vi "Field_C action on update.vi"(4 "Overall status in":T4) -> (0 "Overall status Out":T4, 1 "Command out":T3=enum."Set field")   [LabVIEW 2024, in "Magnet module.lvlib"]
doc: "Evaluates next state machine action at the end of regular check.\nIf field is not at desired value, but reached the closest target it sets new target with new ramp."
uses:
  Magnet module.lvlib
  ctl/RampingOutput.ctl
  ctl/Magnet Orders.ctl
  ctl/Magnet mode.ctl
  ctl/Magnet mode public.ctl
  ctl/SetField data.ctl
  ctl/Overall status.ctl
  ctl/Actual magnet state.ctl
  ctl/Magnet config constants.ctl
  <instrlib>/SMS drivers/Public/PSU Status.ctl
  <instrlib>/SMS drivers/Cryogenic Ltd SMSXXX.lvlib
panel:
  out "error out":errorcluster
  in  "Error In":errorcluster
  in  "PSU Status In":T1 {"Trip Current" format="%.3f"; "Trip Field" format="%.4f"; "Voltage" format="%.2f"; "Field Constant" format="%.6f"; "MID Setpoint (T)" format="%.4f"; "MID Setpoint (A)" format="%.3f"; "MAX Setpoint (T)" format="%.4f"; "MAX Setpoint (A)" format="%.3f"; "Heater Voltage" format="%.2f"; "V Limit (V)" format="%.2f"; "Ramp Rate (A/s)" format="%.3f"; "Output (A)" format="%.3f"; "Output (T)" format="%.4f"; "Persistent Current" format="%.3f"; "Persistent Field" format="%.4f"}
  in  "Magnet Config Constants":T2={"Switch resistant [K]"=5.0, "Switch superconducting [K]"=4.0, "First stage critical temperature [K]"=50.0, "Second stage critical temperature [K]"=5.0, "Inner magnet critical temperature [K]"=6.0, "Outer magnet critical temperature [K]"=5.0, "Field Constant [T/A]"=0.14911, "Maximum Current [A]"=107.3, "Maximum field [T]"=16.0, "Maximum source ramp [A/s]"=0.5, "Source precision [T]"=2e-05, "Ramp limits [A/s]"=[0.0506, 0.038, 0.0285, 0.0213, 0.0104], "Field limits [T]"=[3.0, 9.6, 13.3, 15.5, 16.0], "SMS"="", "LSC218"=""}
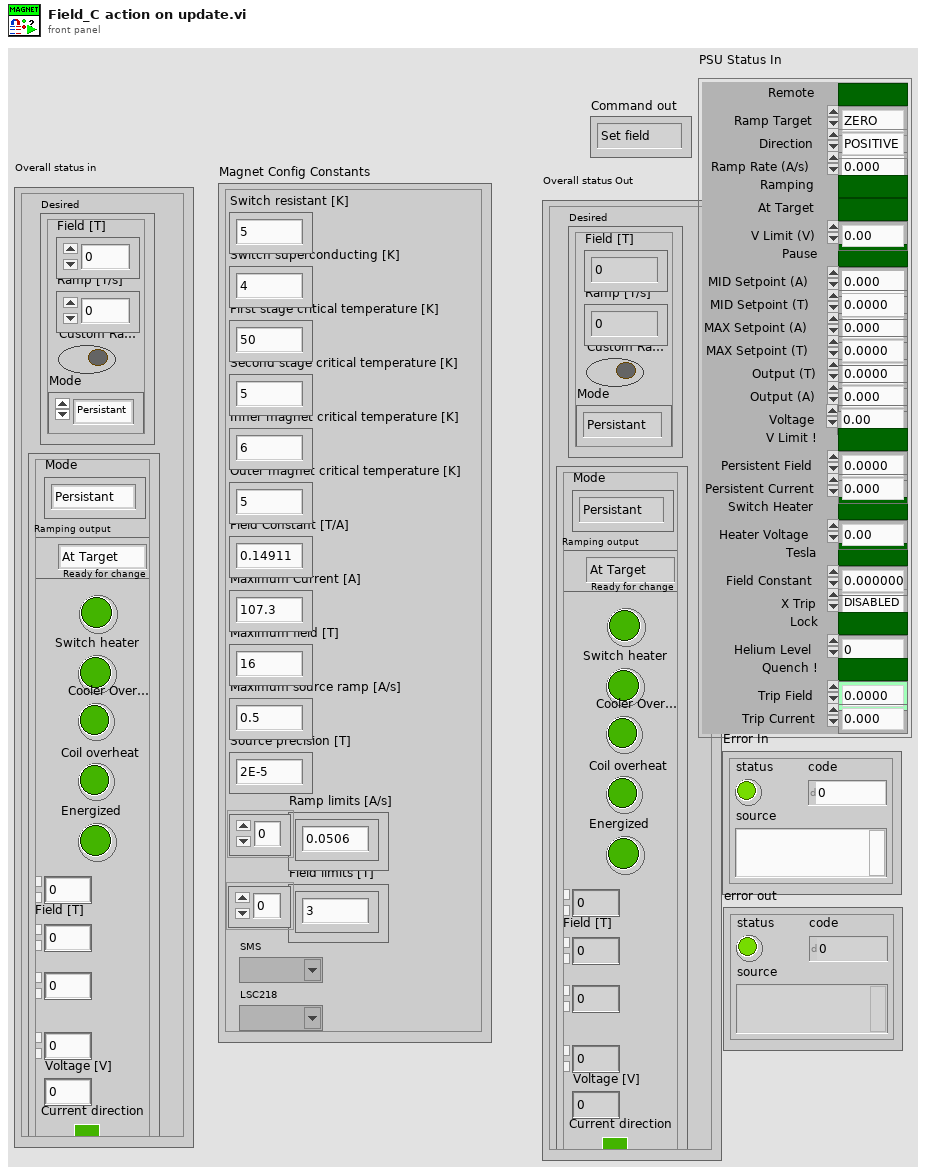
[diagram p1: front panel]
types:
  T1 = typedef "Cryogenic Ltd SMSXXX.lvlib/PSU Status.ctl" = cluster{"Ramp Target":enum16{"ZERO", "MID", "MAX"}, "Pause":bool, "Switch Heater":bool, "Persistent Field":dbl, "Persistent Current":dbl, "Tesla":bool, "Output (T)":dbl, "Output (A)":dbl, "X Trip":enum16{"DISABLED", "ENABLED", "ACTIVE"}, "Ramp Rate (A/s)":dbl, "V Limit (V)":dbl, "Heater Voltage":dbl, "MAX Setpoint (A)":dbl, "MAX Setpoint (T)":dbl, "MID Setpoint (A)":dbl, "MID Setpoint (T)":dbl, "Lock":bool, "Field Constant":dbl, "Remote":bool, "Direction":enum16{"POSITIVE", "NEGATIVE", "OPEN", "UNIPOLAR"}, "Helium Level":u16, "Quench !":bool, "Voltage":dbl, "V Limit !":bool, "Ramping":bool, "At Target":bool, "Trip Field":dbl, "Trip Current":dbl}
  T2 = typedef "Magnet module.lvlib/Magnet config constants.ctl" = cluster{"Switch resistant [K]":dbl, "Switch superconducting [K]":dbl, "First stage critical temperature [K]":dbl, "Second stage critical temperature [K]":dbl, "Inner magnet critical temperature [K]":dbl, "Outer magnet critical temperature [K]":dbl, "Field Constant [T/A]":dbl, "Maximum Current [A]":dbl, "Maximum field [T]":dbl, "Maximum source ramp [A/s]":dbl, "Source precision [T]":dbl, "Ramp limits [A/s]":dbl[], "Field limits [T]":dbl[], "SMS":refnum<visa-resource-name>, "LSC218":refnum<visa-resource-name>}
  T3 = typedef "Magnet module.lvlib/Magnet Orders.ctl" = enum16{"Ignore", "Connect", "Update", "Switch mode", "Set field", "Stop ramping", "Equalize output", "Zero output", "Flip polarity", "Blackout", "Set timer", "Eval temperatures", "Disconnect"}
  T4 = typedef "Magnet module.lvlib/Overall status.ctl" = cluster{"Desired":T5, "Actual":T7}
  T5 = typedef "Magnet module.lvlib/SetField data.ctl" = cluster{"Field [T]":dbl, "Ramp [T/s]":dbl, "Custom Ramp?":bool, "Mode":T6}
  T6 = typedef "Magnet module.lvlib/Magnet mode public.ctl" = enum16{"Persistant", "Ramping"}
  T7 = typedef "Magnet module.lvlib/Actual magnet state.ctl" = cluster{"Mode":T8, "Ramping output":T9, "Ready for change":bool, "Switch heater":bool, "Cooler Overheat":bool, "Coil overheat":bool, "Energized":bool, "Output [T]":dbl, "Field [T]":dbl, "Ramp[T/s]":dbl, "Switch\ntemperature [K]":dbl, "Voltage [V]":dbl, "Current direction":bool}
  T8 = typedef "Magnet module.lvlib/Magnet mode.ctl" = enum16{"Persistant", "Switching", "Ramping", "Quenched"}
  T9 = typedef "Magnet module.lvlib/RampingOutput.ctl" = enum16{"At Target", "Go up", "Go down"}
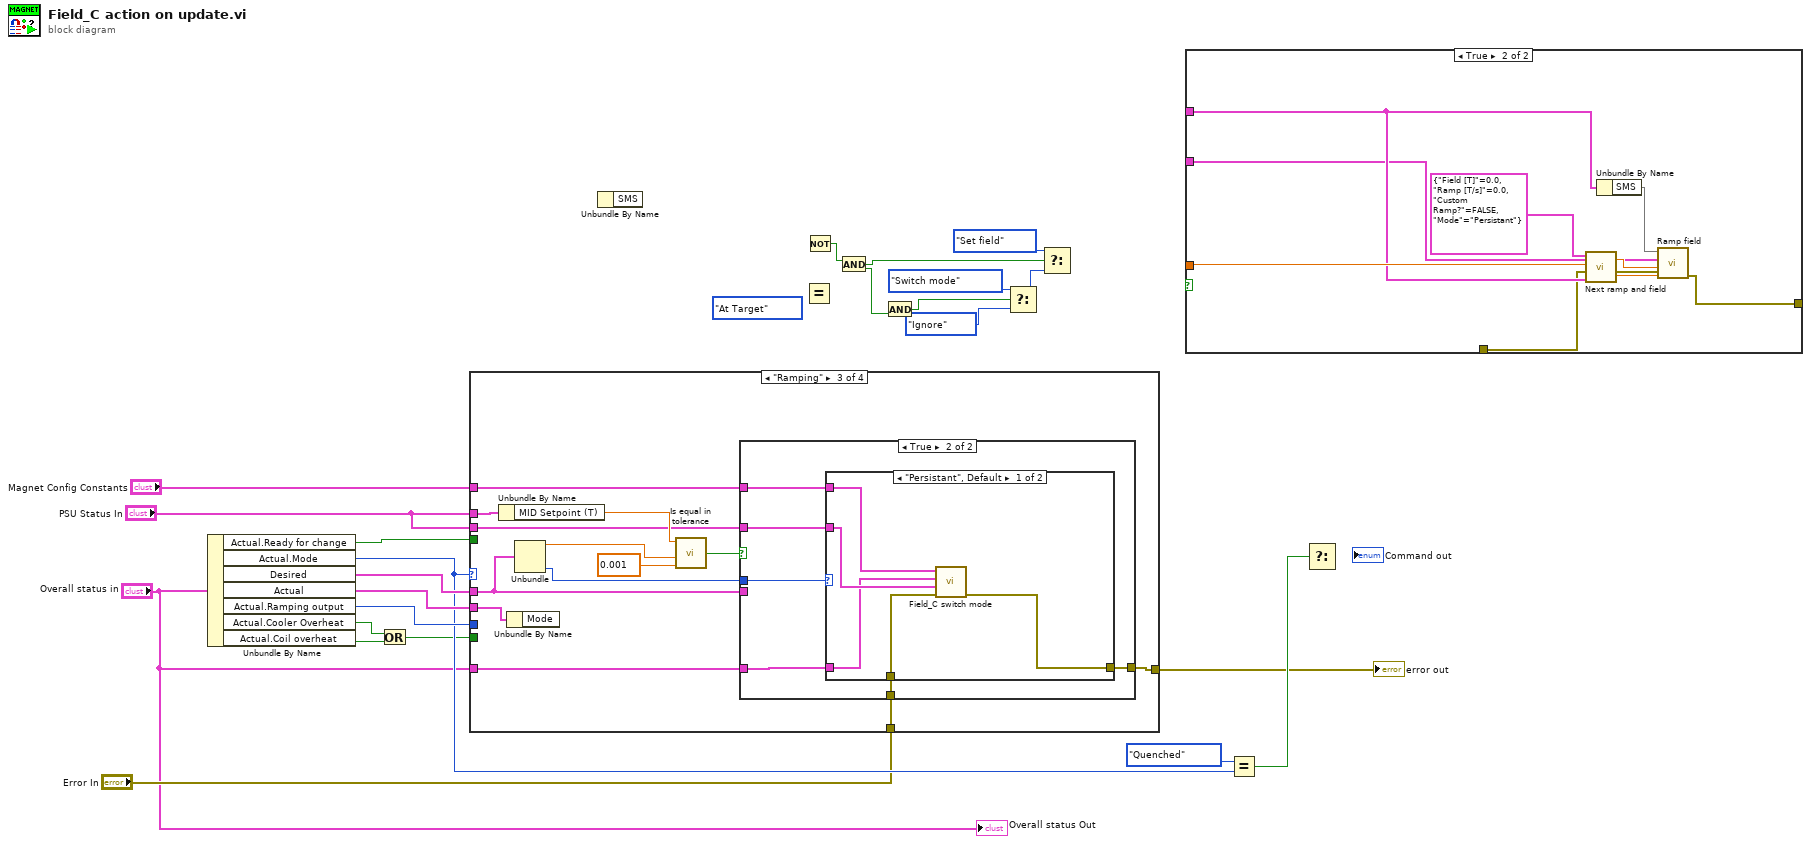
[diagram p0: block diagram]
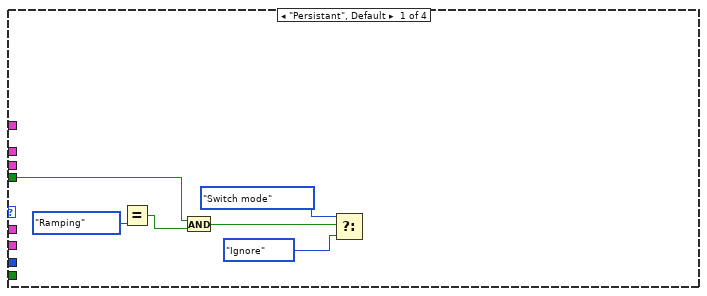
[diagram p3: hidden frame]
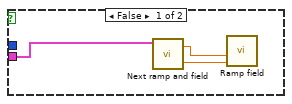
[diagram p5: hidden frame]
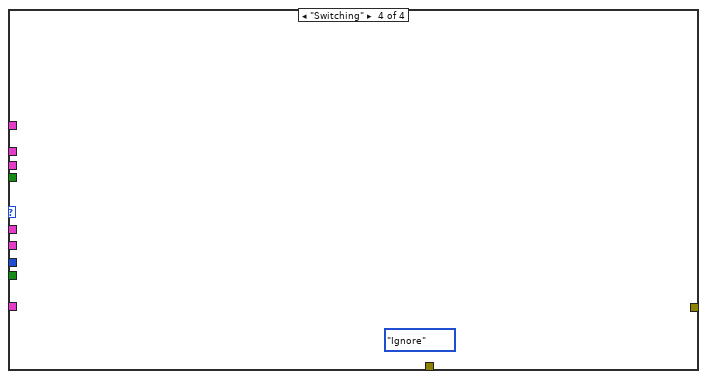
[diagram p7: hidden frame]
diagram:
  (unwired) RampingOutput."At Target" ("x")
  n1 = Unbundle By Name("Overall status in") -> ("Actual.Ready for change"=w15:bool, "Actual.Mode"=w20:T8, "Desired"=w22:T5, "Actual"=w23:T7, "Actual.Ramping output"=w21:T9, "Actual.Cooler Overheat"=w17:bool, "Actual.Coil overheat"=w16:bool)
  n2 = Or(x=w17, y=w16) -> (x .or. y?=w14:bool)
  n3 = case shown="\"Ramping\"" w20 {
    tunnel: w23 -> [_ _ w40 _]
    tunnel: w22 -> [_ _ w41 _]
    tunnel: w21 -> [_ _ _ _]
    tunnel: w15 -> [w24 _ _ _]
    tunnel: w14 -> [_ _ _ _]
    tunnel: "Magnet Config Constants" -> [_ _ w37 _]
    tunnel: "PSU Status In" -> [_ _ w36 _]
    tunnel: [_ _ w33 _] -> w4
    tunnel: "Error In" -> [_ _ w34 _]
    tunnel: "PSU Status In" -> [_ _ w35 _]
    tunnel: "Overall status in" -> [_ _ w32 _]
    frame "Persistant", Default {
      n4 = Equal?(y=Magnet_mode_public."Ramping" ("Mode")) -> (x=w27:T6, x = y?=w25:bool)
      n5 = And(x=w24, y=w25) -> (x .and. y?=w28:bool)
      n6 = Select(t=Magnet_Orders."Switch mode" ("Command out"), s=w28, f=Magnet_Orders."Ignore" ("Command out")) -> (s? t:f=w29:T3)
    }
    frame "Quenched" {
      # "If quenched, do nothing or just set current to zero"
    }
    frame "Ramping" {
      n7 = Unbundle By Name(w36) -> ("MID Setpoint (T)"=w43:dbl)
      n8 = Unbundle By Name(w40) -> ()  [unwired: 1 out]
      n9 = Unbundle(w41) -> ("Field [T]"=w42:dbl, "Mode"=w38:T6)  [unwired: 2 out]
      n10 = call "Is equal in tolerance.vi"("Absolut tolerance"=0.001, "Reference value"=w42, "Input value"=w43) -> ("Is in range"=w39:bool)  [unwired: 1 in]
      n11 = case shown="True" w39 {
        tunnel: w41 -> [w45 _]
        tunnel: w38 -> [_ w53]
        tunnel: w37 -> [_ w52]
        tunnel: w35 -> [_ w51]
        tunnel: w34 -> [_ w50]
        tunnel: [_ w49] -> w33
        tunnel: w32 -> [_ w48]
        frame False {
          n12 = call "Next ramp and field.vi"("Desired"=w45) -> ("Ramp to set [A/s]"=w47:dbl, "Field to set [T]"=w46:dbl)  [unwired: 3 in]
          n13 = call "Ramp field.vi"("Ramp to set [A/s]"=w47, "Field to set [T]"=w46) -> ()  [unwired: 6 in, 4 out]
        }
        frame True {
          n14 = case shown="\"Persistant\", Default" w53 {
            tunnel: w52 -> [w54 _]
            tunnel: w51 -> [w58 _]
            tunnel: w50 -> [w57 _]
            tunnel: [w56 _] -> w49
            tunnel: w48 -> [w55 _]
            frame "Persistant", Default {
              n15 = call "Field_C switch mode.vi"("error in (no error)"=w57, "PSU Status"=w58, "Overall status in"=w55, "Magnet Constants"=w54) -> ("error out"=w56:errorcluster)  [unwired: 5 in, 2 out]
            }
            frame "Ramping" {
            }
          }
        }
      }
    }
    frame "Switching" {
      (unwired) Magnet_Orders."Ignore" ("Command out")
    }
  }
  "error out" <- w4
  n16 = Unbundle By Name() -> ()  [unwired: 1 in, 1 out]
  n17 = Equal?() -> ()  [unwired: 2 in, 1 out]
  n18 = Not() -> (.not. x?=w9:bool)  [unwired: 1 in]
  n19 = And(x=w9) -> (y=w13:bool, x .and. y?=w10:bool)
  n20 = And(y=w13) -> (x .and. y?=w12:bool)  [unwired: 1 in]
  n21 = Select(t=Magnet_Orders."Switch mode", s=w12, f=Magnet_Orders."Ignore" ("Command out")) -> (s? t:f=w11:T3)
  n22 = Select(t=Magnet_Orders."Set field" ("Command out"), s=w10, f=w11) -> ()  [unwired: 1 out]
  n23 = case shown="True" {
    selector: _ -> [_ _]
    tunnel: _ -> [_ w66]
    tunnel: _ -> [_ w64]
    tunnel: _ -> [_ w62]
    tunnel: [w59 w60] -> _
    tunnel: [w59 w61] -> _
    frame False {
    }
    frame True {
      n24 = call "Next ramp and field.vi"("Magnet Constants in"=w64, "Actual field [T]"=w66, "Desired"=T5 {"Field [T]"=0.0, "Ramp [T/s]"=0.0, "Custom Ramp?"=FALSE, "Mode"=enum."Persistant"}) -> ("Ramp to set [A/s]"=w67:dbl, "Field to set [T]"=w68:dbl)  [unwired: 1 in]
      n25 = Unbundle By Name(w64) -> ("SMS"=w63)
      n26 = call "Ramp field.vi"("Ramp to set [A/s]"=w67, "Field to set [T]"=w68, "PSU Status In"=w62, "VISA Refnum in"=w63) -> ("error out"=w60:errorcluster, "Error In"=w61:errorcluster)  [unwired: 3 in, 3 out]
    }
  }
  n27 = Equal?(x=Magnet_mode."Quenched", y=w20) -> (x = y?=w18:bool)
  n28 = Select(s=w18) -> ()  [unwired: 2 in, 1 out]
  "Overall status Out" <- "Overall status in"
